vi "telem.vi"() -> ()   [LabVIEW 2015]
uses:
  <vilib>/Instr/_visa.llb/VISA Configure Serial Port (Instr).vi
panel:
  out "Heartbeat":bool
  in  "?":T1(tab)
  out "Pack voltage":u8(slide) scale=80.0..126.0
  out "Pack current":dbl format="%#_4gA"
  out "Max temperature":dbl format="%#_g°C"
  out "Pack voltage":dbl format="%#_5gV"
  out "Max voltage":dbl format="%#_4gV"
  out "Min voltage":dbl format="%#_4gV"
  in  "COM port":refnum<visa-resource-name>
  out "Battery status":bool
  out "Motor current":dbl format="%#_3fA"
  out "Battery status":bool
  out "Pack current":dbl format="%#_4gA"
  out "Temperature":u8[](array[numeric]) format="%d°C"
  out "Max temperature":dbl format="%#_g°C"
  out "Pack voltage":dbl format="%#_5gV"
  out "Max voltage":dbl format="%#_4gV"
  out "Min voltage":dbl format="%#_4gV"
  out "Voltage":u16[](array[slide]) scale=107.0..164.0
  out "Voltage":dbl[][](array[numeric]) format="%#_4gV"
  out "State of charge":dbl[][](array[numeric]) format="%#_4g%"
  out "Discharge":bool[](array[boolean])
  out "Motor power consumption":dbl format="%#_3fW"
  out "Gauge":dbl(knob) scale=0.0..100.0
  out "Motor velocity":dbl format="%#_7fkm/h"
  out "Bus voltage":dbl format="%#_3fV"
  out "Motor current":dbl format="%#_3fA"
  out "Motor rpm":dbl format="%#_10frpm"
  out "Motor internal temperature":dbl format="%#_3f°C"
  out "Motor heatsink temperature":dbl format="%#_3f°C"
  out "DSP board temperature":dbl format="%#_3f°C"
  out "Desired rpm":dbl format="%#_3frpm"
  out "Throttle":dbl format="%#_3f%"
  out "Array 1":bool[](array[boolean])
  out "Vin (1)":dbl format="%.2f"
  out "Vout (1)":dbl format="%.2f"
  out "Array 2":bool[](array[boolean])
  out "Array 3":bool[](array[boolean])
  out "Vin (3)":dbl format="%.2f"
  out "Vout (3)":dbl format="%.2f"
  out "Array 4":bool[](array[boolean])
  out "Vin (4)":dbl format="%.2f"
  out "Vout (4)":dbl format="%.2f"
  out "Iin (1)":dbl format="%.2f"
  out "Temperature (1)":u8
  out "Vin (2)":dbl
  out "Vout (2)":dbl format="%.2f"
  out "Iin (3)":dbl format="%.2f"
  out "Temperature (3)":u8
  out "Iin (4)":dbl format="%.2f"
  out "Temperature (4)":u8
  out "Iin (2)":dbl format="%.2f"
  out "Temperature (2)":u8
  out "Aux voltage":dbl
  out "DC/DC converter temperature":dbl format="%#_3g"
  out "Array connected":bool
  out "Motor connected":bool
  out "Aux cell voltages":dbl[][](array[numeric]) format="%#_4gV"
  out "0x0B - BPS voltage":string
  out "0x07 - Motor heatsink temperature":string
  out "0x05 - Motor velocity":string
  out "0x03 - Motor bus vi":string
  out "0x0D - BPS temperature":string
  out "0x11 - BPS current, balancing, status":string
  out "0x1D - MPPT":string
  out "0x09 - Motor DSP temperature":string
  out "0x19 - PMS data":string
  out "0x0A - EVDC drive":string
  # "1         2         3        4         5         6           7        8        9         10       11       12       13       14       15       16       17       18        19      20       21        22       23      24       25       26      27        28       29        30"
  # "UNDV  |  NOC   |  OVT  | BVLR"
  # "UNDV  |  NOC   |  OVT  | BVLR"
  # "UNDV  |  NOC   |  OVT  | BVLR"
  # "UNDV  |  NOC   |  OVT  | BVLR"
  # "Cell 1   |   Cell 2   |   Cell 3  |    Cell 4"
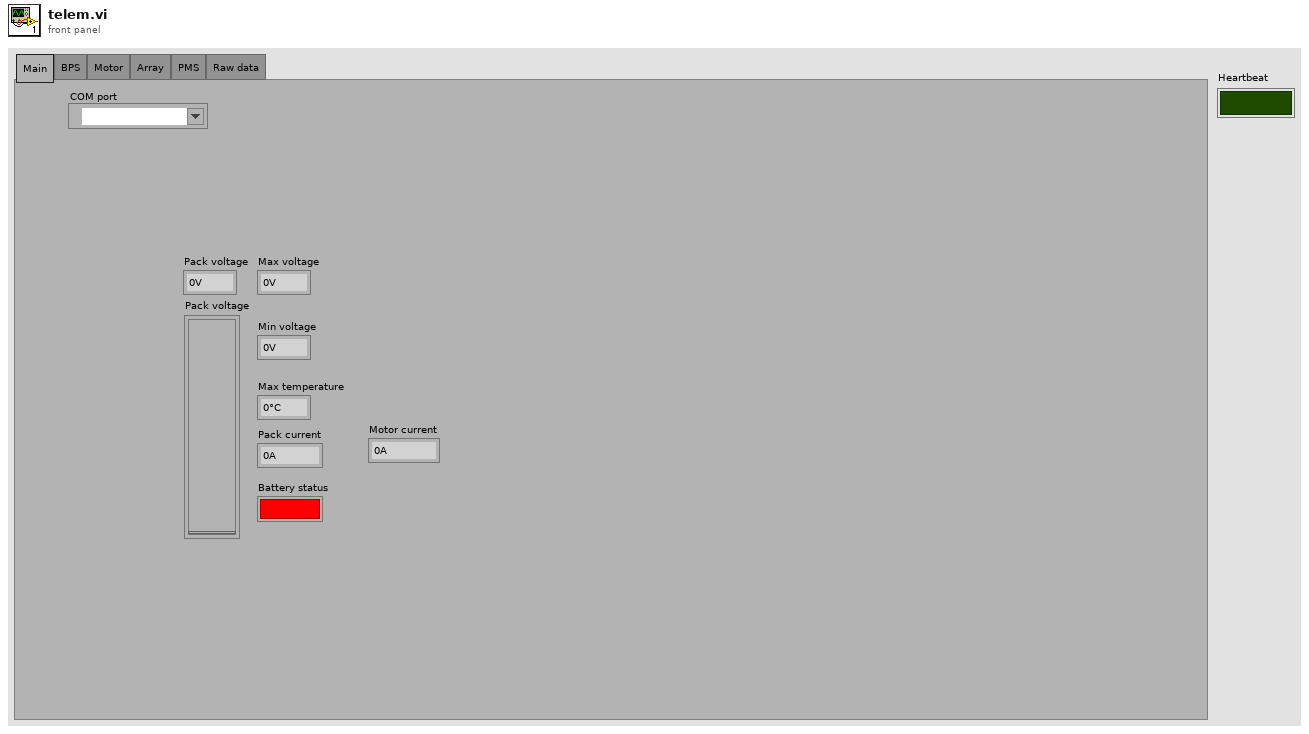
[diagram p1: front panel]
types:
  T1 = enum32{"Main", "BPS", "Motor", "Array", "PMS", "Raw data"}
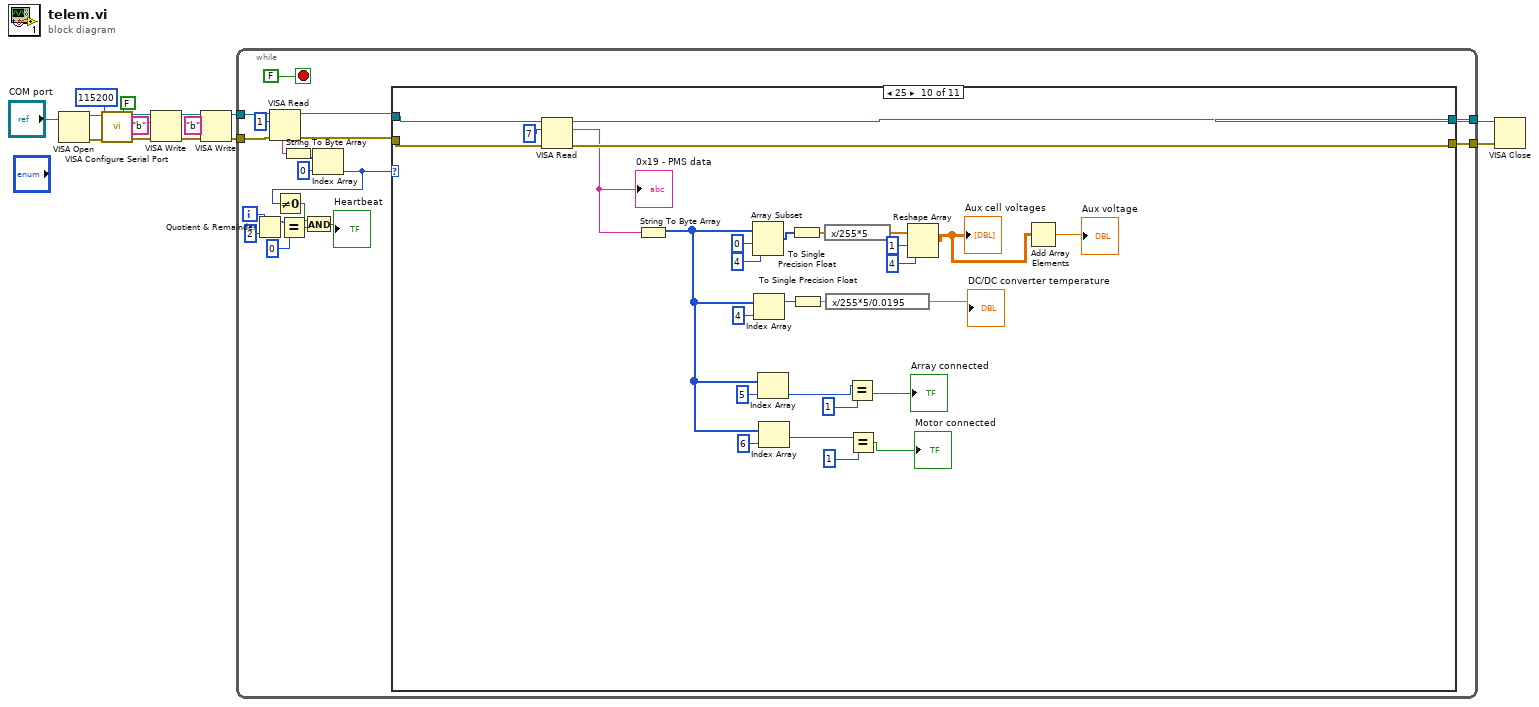
[diagram p0: block diagram]
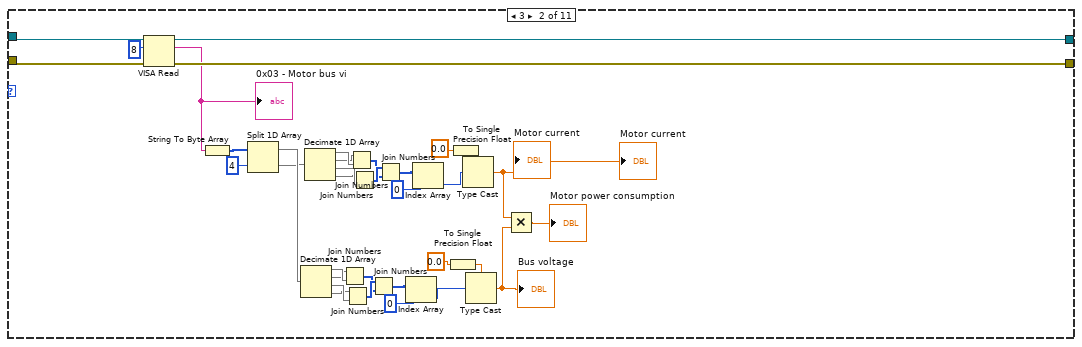
[diagram p3: hidden frame]
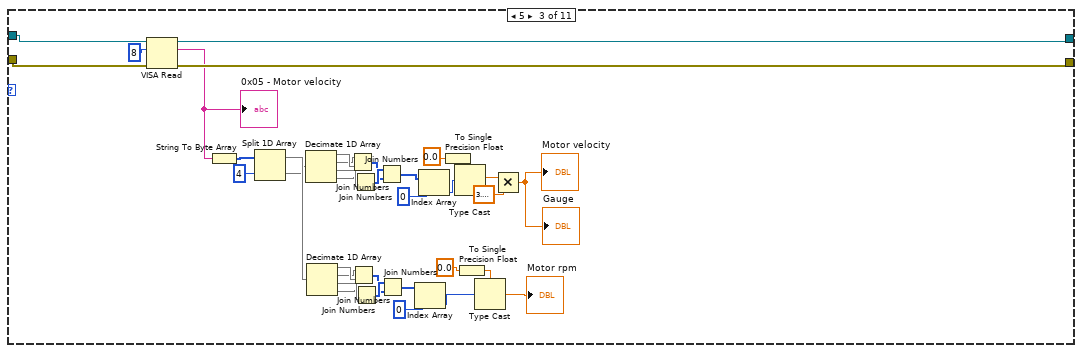
[diagram p4: hidden frame]
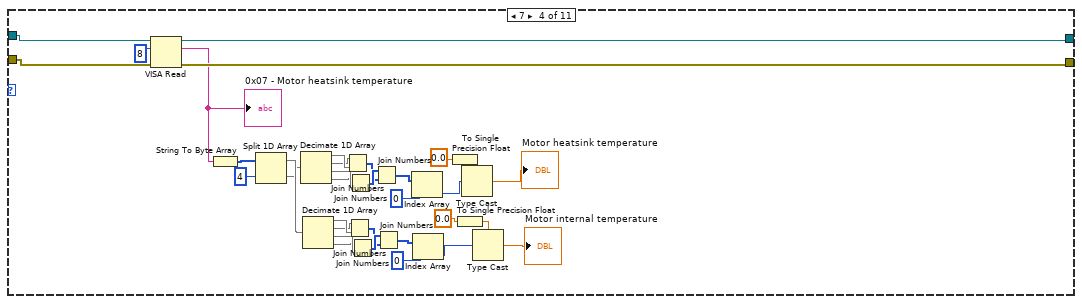
[diagram p5: hidden frame]
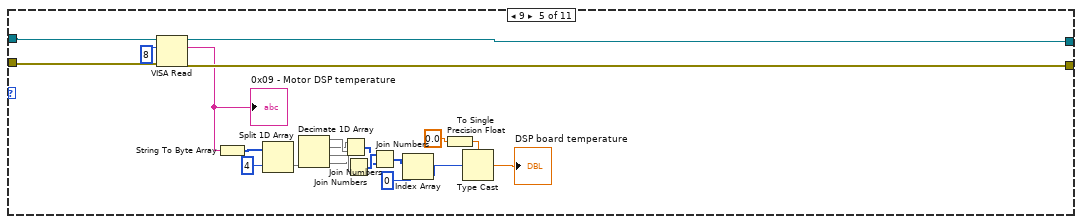
[diagram p6: hidden frame]
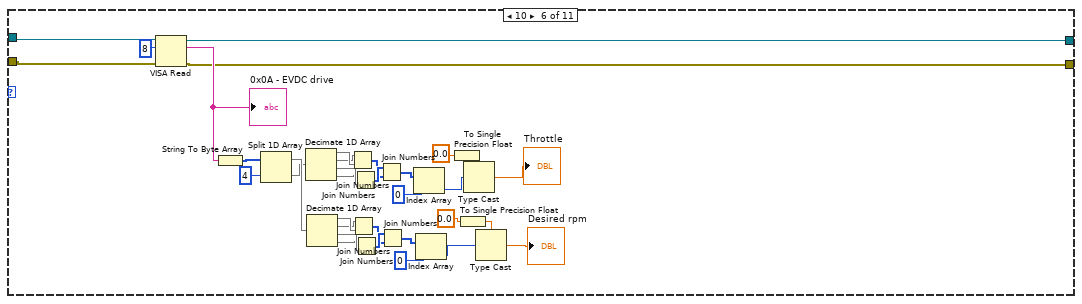
[diagram p7: hidden frame]
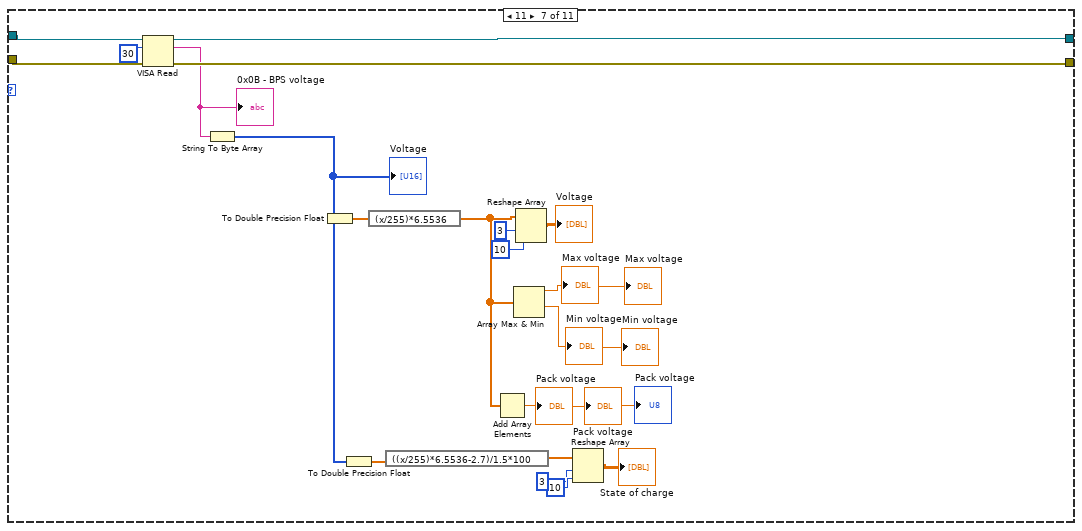
[diagram p8: hidden frame]
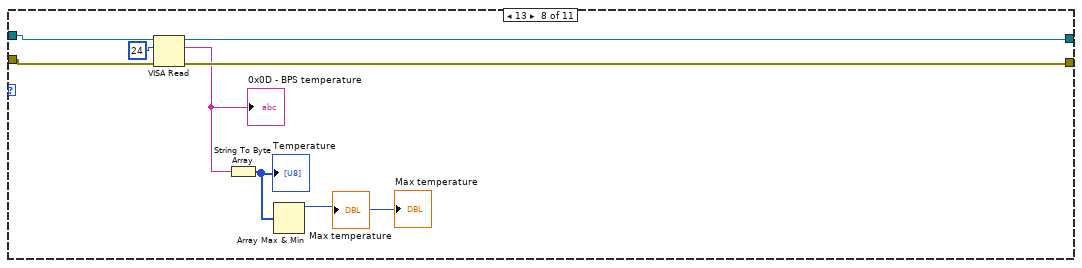
[diagram p9: hidden frame]
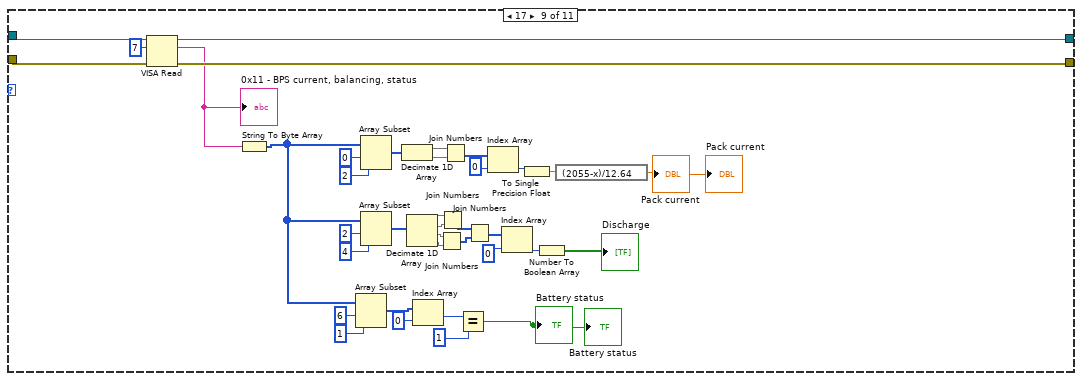
[diagram p10: hidden frame]
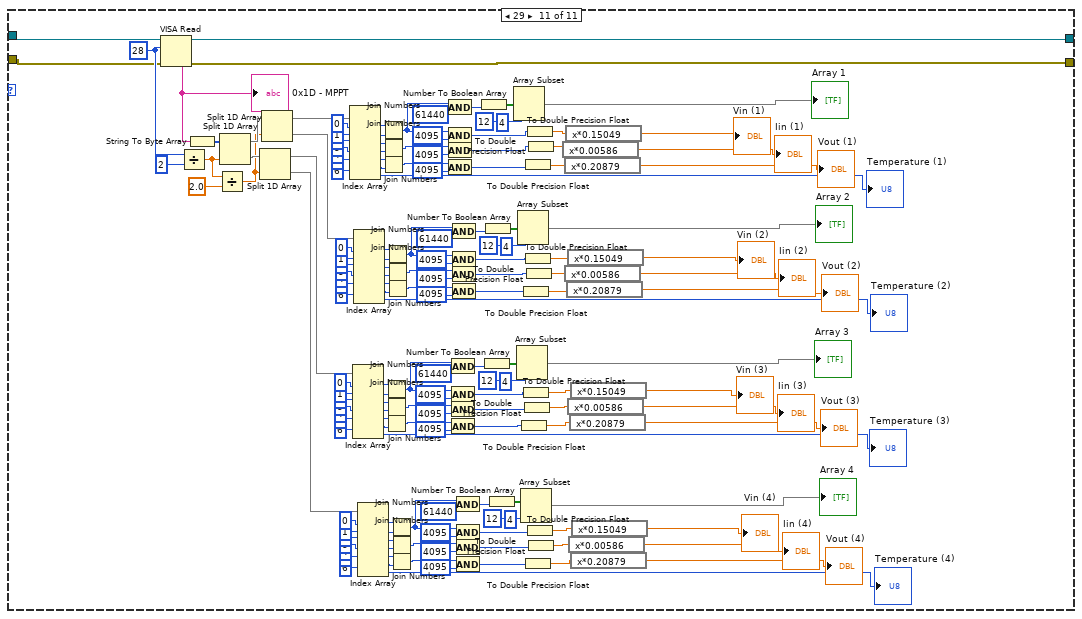
[diagram p11: hidden frame]
diagram:
  n1 = VISA Open(VISA resource name="COM port") -> (VISA resource name=w15:refnum<visa-resource-name>, error out=w14:errorcluster)  [unwired: 4 in]
  n2 = call-poly "VISA Configure Serial Port"("VISA resource name"=w15, "Enable Termination\nChar (T)"=FALSE ("Enable Termination\nChar (T)"), "baud rate (9600)"=u32 115200, "error in (no error)"=w14) -> ("VISA resource name out"=w8:refnum<visa-resource-name>, "error out"=w7:errorcluster)  [unwired: 10 in]
  n3 = VISA Write(VISA resource name=w8, write buffer="b", error in (no error)=w7) -> (VISA resource name out=w10:refnum<visa-resource-name>, error out=w9:errorcluster)  [unwired: 1 out]
  n4 = VISA Write(VISA resource name=w10, write buffer="b", error in (no error)=w9) -> (VISA resource name out=w3:refnum<visa-resource-name>, error out=w2:errorcluster)  [unwired: 1 out]
  n5 = while {
    tunnel: [w28] -> w5
    tunnel: [w27] -> w4
    tunnel: w3 -> [w17]
    tunnel: w2 -> [w16]
    i -> [w25]
    stop <- FALSE stop-if-true
    n6 = Quotient & Remainder(x=w25, y=2) -> (x-y*floor(x/y)=w23:i32)  [unwired: 1 out]
    n7 = VISA Read(VISA resource name=w17, byte count=u32 1, error in (no error)=w16) -> (VISA resource name out=w30:refnum<visa-resource-name>, read buffer=w33:string, error out=w29:errorcluster)  [unwired: 1 out]
    n8 = Equal?(x=w23, y=0) -> (x = y?=w21:bool)
    n9 = String To Byte Array(string=w33) -> (unsigned byte array=w32:u8[])
    n10 = Index Array(array=w32, index=0) -> (element=w18:u8)
    n11 = Not Equal To 0?(x=w18) -> (x != 0?=w20:bool)
    n12 = And(x=w20, y=w21) -> (x .and. y?=→"Heartbeat":bool)
    n13 = case shown="25" w18 {
      tunnel: w30 -> [w36 w53 w89 w125 w151 w180 w199 w218 w250 w286 w331]
      tunnel: w29 -> [w35 w52 w88 w124 w150 w179 w198 w217 w249 w285 w330]
      tunnel: [w36 w71 w107 w141 w162 w183 w216 w224 w261 w289 w446] -> w28
      tunnel: [w35 w70 w106 w140 w161 w182 w215 w223 w260 w288 w445] -> w27
      frame Default {
      }
      frame 3 {
        n14 = VISA Read(VISA resource name=w53, byte count=u32 8, error in (no error)=w52) -> (VISA resource name out=w71:refnum<visa-resource-name>, read buffer=w69:string, error out=w70:errorcluster)  [unwired: 1 out]
        "0x03 - Motor bus vi" <- w69
        n15 = String To Byte Array(string=w69) -> (unsigned byte array=w68:u8[])
        n16 = Split 1D Array(array=w68, index=4) -> (first subarray=w39:u8[], second subarray=w38:u8[])
        n17 = Decimate 1D Array(w39) -> (w41:u8[], w40:u8[], w43:u8[], w42:u8[])
        n18 = Decimate 1D Array(w38) -> (w51:u8[], w50:u8[], w49:u8[], w48:u8[])
        n19 = Join Numbers(hi=w40, lo=w41) -> ((hi.lo)=w44:u16[])
        n20 = Join Numbers(hi=w42, lo=w43) -> ((hi.lo)=w45:u16[])
        n21 = Join Numbers(hi=w50, lo=w51) -> ((hi.lo)=w46:u16[])
        n22 = Join Numbers(hi=w48, lo=w49) -> ((hi.lo)=w47:u16[])
        n23 = Join Numbers(hi=w45, lo=w44) -> ((hi.lo)=w64:u32[])
        n24 = Join Numbers(hi=w47, lo=w46) -> ((hi.lo)=w66:u32[])
        n25 = Index Array(array=w64, index=0) -> (element=w58:u32)
        n26 = Index Array(array=w66, index=0) -> (element=w62:u32)
        n27 = To Single Precision Float(number=sgl 0.0) -> (single precision float=w59:sgl)
        n28 = To Single Precision Float(number=sgl 0.0) -> (single precision float=w61:sgl)
        n29 = Type Cast(type=w61, x=w62) -> (*(type *) &x=w37:sgl)
        "Motor current" <- w37
        "Motor current" <- w37
        n30 = Type Cast(type=w59, x=w58) -> (*(type *) &x=w56:sgl)
        "Bus voltage" <- w56
        n31 = Multiply(x=w37, y=w56) -> (x*y=→"Motor power consumption":sgl)
      }
      frame 5 {
        n32 = VISA Read(VISA resource name=w89, byte count=u32 8, error in (no error)=w88) -> (VISA resource name out=w107:refnum<visa-resource-name>, read buffer=w94:string, error out=w106:errorcluster)  [unwired: 1 out]
        "0x05 - Motor velocity" <- w94
        n33 = String To Byte Array(string=w94) -> (unsigned byte array=w105:u8[])
        n34 = Split 1D Array(array=w105, index=4) -> (first subarray=w73:u8[], second subarray=w72:u8[])
        n35 = Decimate 1D Array(w72) -> (w87:u8[], w86:u8[], w85:u8[], w84:u8[])
        n36 = Decimate 1D Array(w73) -> (w81:u8[], w80:u8[], w79:u8[], w78:u8[])
        n37 = Join Numbers(hi=w86, lo=w87) -> ((hi.lo)=w82:u16[])
        n38 = Join Numbers(hi=w80, lo=w81) -> ((hi.lo)=w76:u16[])
        n39 = Join Numbers(hi=w84, lo=w85) -> ((hi.lo)=w83:u16[])
        n40 = Join Numbers(hi=w78, lo=w79) -> ((hi.lo)=w77:u16[])
        n41 = Join Numbers(hi=w83, lo=w82) -> ((hi.lo)=w74:u32[])
        n42 = Join Numbers(hi=w77, lo=w76) -> ((hi.lo)=w75:u32[])
        n43 = Index Array(array=w75, index=0) -> (element=w97:u32)
        n44 = Index Array(array=w74, index=0) -> (element=w101:u32)
        n45 = To Single Precision Float(number=sgl 0.0) -> (single precision float=w100:sgl)
        n46 = Type Cast(type=w100, x=w101) -> (*(type *) &x=w93:sgl)
        n47 = To Single Precision Float(number=sgl 0.0) -> (single precision float=w98:sgl)
        n48 = Type Cast(type=w98, x=w97) -> (*(type *) &x=→"Motor rpm":sgl)
        n49 = Multiply(x=w93, y=sgl 3.6) -> (x*y=→"Motor velocity" →"Gauge":sgl)
      }
      frame 7 {
        n50 = VISA Read(VISA resource name=w125, byte count=u32 8, error in (no error)=w124) -> (VISA resource name out=w141:refnum<visa-resource-name>, read buffer=w127:string, error out=w140:errorcluster)  [unwired: 1 out]
        "0x07 - Motor heatsink temperature" <- w127
        n51 = String To Byte Array(string=w127) -> (unsigned byte array=w139:u8[])
        n52 = Split 1D Array(array=w139, index=4) -> (first subarray=w109:u8[], second subarray=w108:u8[])
        n53 = Decimate 1D Array(w108) -> (w123:u8[], w122:u8[], w121:u8[], w120:u8[])
        n54 = Decimate 1D Array(w109) -> (w116:u8[], w115:u8[], w114:u8[], w113:u8[])
        n55 = Join Numbers(hi=w122, lo=w123) -> ((hi.lo)=w118:u16[])
        n56 = Join Numbers(hi=w115, lo=w116) -> ((hi.lo)=w111:u16[])
        n57 = Join Numbers(hi=w120, lo=w121) -> ((hi.lo)=w119:u16[])
        n58 = Join Numbers(hi=w113, lo=w114) -> ((hi.lo)=w112:u16[])
        n59 = Join Numbers(hi=w119, lo=w118) -> ((hi.lo)=w117:u32[])
        n60 = Join Numbers(hi=w112, lo=w111) -> ((hi.lo)=w110:u32[])
        n61 = Index Array(array=w117, index=0) -> (element=w135:u32)
        n62 = Index Array(array=w110, index=0) -> (element=w130:u32)
        n63 = To Single Precision Float(number=sgl 0.0) -> (single precision float=w133:sgl)
        n64 = To Single Precision Float(number=sgl 0.0) -> (single precision float=w131:sgl)
        n65 = Type Cast(type=w133, x=w135) -> (*(type *) &x=→"Motor heatsink temperature":sgl)
        n66 = Type Cast(type=w131, x=w130) -> (*(type *) &x=→"Motor internal temperature":sgl)
      }
      frame 9 {
        n67 = VISA Read(VISA resource name=w151, byte count=u32 8, error in (no error)=w150) -> (VISA resource name out=w162:refnum<visa-resource-name>, read buffer=w153:string, error out=w161:errorcluster)  [unwired: 1 out]
        "0x09 - Motor DSP temperature" <- w153
        n68 = String To Byte Array(string=w153) -> (unsigned byte array=w160:u8[])
        n69 = Split 1D Array(array=w160, index=4) -> (second subarray=w142:u8[])  [unwired: 1 out]
        n70 = Decimate 1D Array(w142) -> (w149:u8[], w148:u8[], w147:u8[], w146:u8[])
        n71 = Join Numbers(hi=w148, lo=w149) -> ((hi.lo)=w144:u16[])
        n72 = Join Numbers(hi=w146, lo=w147) -> ((hi.lo)=w145:u16[])
        n73 = Join Numbers(hi=w145, lo=w144) -> ((hi.lo)=w143:u32[])
        n74 = Index Array(array=w143, index=0) -> (element=w156:u32)
        n75 = To Single Precision Float(number=sgl 0.0) -> (single precision float=w157:sgl)
        n76 = Type Cast(type=w157, x=w156) -> (*(type *) &x=→"DSP board temperature":sgl)
      }
      frame 10 {
        n77 = VISA Read(VISA resource name=w180, byte count=u32 8, error in (no error)=w179) -> (VISA resource name out=w183:refnum<visa-resource-name>, read buffer=w184:string, error out=w182:errorcluster)  [unwired: 1 out]
        "0x0A - EVDC drive" <- w184
        n78 = String To Byte Array(string=w184) -> (unsigned byte array=w196:u8[])
        n79 = Split 1D Array(array=w196, index=4) -> (first subarray=w164:u8[], second subarray=w163:u8[])
        n80 = Decimate 1D Array(w163) -> (w178:u8[], w177:u8[], w176:u8[], w175:u8[])
        n81 = Decimate 1D Array(w164) -> (w172:u8[], w171:u8[], w170:u8[], w169:u8[])
        n82 = Join Numbers(hi=w177, lo=w178) -> ((hi.lo)=w173:u16[])
        n83 = Join Numbers(hi=w171, lo=w172) -> ((hi.lo)=w167:u16[])
        n84 = Join Numbers(hi=w175, lo=w176) -> ((hi.lo)=w174:u16[])
        n85 = Join Numbers(hi=w169, lo=w170) -> ((hi.lo)=w168:u16[])
        n86 = Join Numbers(hi=w174, lo=w173) -> ((hi.lo)=w165:u32[])
        n87 = Join Numbers(hi=w168, lo=w167) -> ((hi.lo)=w166:u32[])
        n88 = Index Array(array=w165, index=0) -> (element=w192:u32)
        n89 = Index Array(array=w166, index=0) -> (element=w187:u32)
        n90 = To Single Precision Float(number=sgl 0.0) -> (single precision float=w190:sgl)
        n91 = To Single Precision Float(number=sgl 0.0) -> (single precision float=w188:sgl)
        n92 = Type Cast(type=w190, x=w192) -> (*(type *) &x=→"Throttle":sgl)
        n93 = Type Cast(type=w188, x=w187) -> (*(type *) &x=→"Desired rpm":sgl)
      }
      frame 11 {
        n94 = VISA Read(VISA resource name=w199, byte count=u32 30, error in (no error)=w198) -> (VISA resource name out=w216:refnum<visa-resource-name>, read buffer=w204:string, error out=w215:errorcluster)  [unwired: 1 out]
        "0x0B - BPS voltage" <- w204
        n95 = String To Byte Array(string=w204) -> (unsigned byte array=w197:u8[])
        "Voltage" <- w197
        n96 = To Double Precision Float(number=w197) -> (double precision float=w214:dbl[])
        n97 = To Double Precision Float(number=w197) -> (double precision float=w213:dbl[])
        n98 = expression code="(x/255)*6.5536"(w214) -> (w205:dbl[])
        n99 = expression code="((x/255)*6.5536-2.7)/1.5*100"(w213) -> (w209:dbl[])
        n100 = Add Array Elements(numeric array=w205) -> (sum=→"Pack voltage" →"Pack voltage" →"Pack voltage":dbl)
        n101 = Array Max & Min(array=w205) -> (max value=→"Max voltage" →"Max voltage":dbl, min value=→"Min voltage" →"Min voltage":dbl)  [unwired: 2 out]
        n102 = Reshape Array(w205, 3 ("dimension size"), 10 ("dimension size")) -> (→"Voltage":dbl[][])
        n103 = Reshape Array(w209, 3 ("dimension size"), 10 ("dimension size")) -> (→"State of charge":dbl[][])
      }
      frame 13 {
        n104 = VISA Read(VISA resource name=w218, byte count=u32 24, error in (no error)=w217) -> (VISA resource name out=w224:refnum<visa-resource-name>, read buffer=w221:string, error out=w223:errorcluster)  [unwired: 1 out]
        "0x0D - BPS temperature" <- w221
        n105 = String To Byte Array(string=w221) -> (unsigned byte array=w222:u8[])
        "Temperature" <- w222
        n106 = Array Max & Min(array=w222) -> (max value=→"Max temperature" →"Max temperature":u8)  [unwired: 3 out]
      }
      frame 17 {
        n107 = VISA Read(VISA resource name=w250, byte count=u32 7, error in (no error)=w249) -> (VISA resource name out=w261:refnum<visa-resource-name>, read buffer=w255:string, error out=w260:errorcluster)  [unwired: 1 out]
        "0x11 - BPS current, balancing, status" <- w255
        n108 = String To Byte Array(string=w255) -> (unsigned byte array=w227:u8[])
        n109 = Array Subset(array=w227, index=6, length=1) -> (w229:u8[])
        n110 = Array Subset(array=w227, index=0, length=2) -> (w246:u8[])
        n111 = Array Subset(array=w227, index=2, length=4) -> (w234:u8[])
        n112 = Decimate 1D Array(w246) -> (w253:u8[], w252:u8[])
        n113 = Decimate 1D Array(w234) -> (w243:u8[], w242:u8[], w241:u8[], w240:u8[])
        n114 = Index Array(array=w229, index=0) -> (element=w233:u8)
        n115 = Join Numbers(hi=w241, lo=w240) -> ((hi.lo)=w239:u16[])
        n116 = Join Numbers(hi=w243, lo=w242) -> ((hi.lo)=w238:u16[])
        n117 = Join Numbers(hi=w253, lo=w252) -> ((hi.lo)=w258:u16[])
        n118 = Equal?(x=w233, y=u16 1) -> (x = y?=→"Battery status" →"Battery status":bool)
        n119 = Join Numbers(hi=w238, lo=w239) -> ((hi.lo)=w244:u32[])
        n120 = Index Array(array=w258, index=0) -> (element=w256:u16)
        n121 = Index Array(array=w244, index=0) -> (element=w245:u32)
        n122 = To Single Precision Float(number=w256) -> (single precision float=w257:sgl)
        n123 = Number To Boolean Array(number=w245) -> (Boolean array=→"Discharge":bool[])
        n124 = expression code="(2055-x)/12.64"(w257) -> (→"Pack current" →"Pack current":sgl)
      }
      frame 25 {
        n125 = VISA Read(VISA resource name=w286, byte count=u32 7, error in (no error)=w285) -> (VISA resource name out=w289:refnum<visa-resource-name>, read buffer=w284:string, error out=w288:errorcluster)  [unwired: 1 out]
        "0x19 - PMS data" <- w284
        n126 = String To Byte Array(string=w284) -> (unsigned byte array=w279:u8[])
        n127 = Array Subset(array=w279, index=0, length=4) -> (w267:u8[])
        n128 = Index Array(array=w279, index=4) -> (element=w265:u8)
        n129 = Index Array(array=w279, index=5) -> (element=w274:u8)
        n130 = Index Array(array=w279, index=6) -> (element=w276:u8)
        n131 = To Single Precision Float(number=w267) -> (single precision float=w268:sgl[])
        n132 = To Single Precision Float(number=w265) -> (single precision float=w266:sgl)
        n133 = expression code="x/255*5"(w268) -> (w269:sgl[])
        n134 = expression code="x/255*5/0.0195"(w266) -> (→"DC/DC converter temperature":sgl)
        n135 = Equal?(x=w274, y=u16 1) -> (x = y?=→"Array connected":bool)
        n136 = Equal?(x=w276, y=u16 1) -> (x = y?=→"Motor connected":bool)
        n137 = Reshape Array(w269, 1 ("dimension size"), 4 ("dimension size")) -> (w263:sgl[][])
        "Aux cell voltages" <- w263
        n138 = Add Array Elements(numeric array=w263) -> (sum=→"Aux voltage":sgl)
      }
      frame 29 {
        w332 = u32 28 ("byte count")
        n139 = VISA Read(VISA resource name=w331, byte count=w332, error in (no error)=w330) -> (VISA resource name out=w446:refnum<visa-resource-name>, read buffer=w444:string, error out=w445:errorcluster)  [unwired: 1 out]
        "0x1D - MPPT" <- w444
        n140 = Divide(x=w332, y=u8 2) -> (x/y=w431:dbl)
        n141 = String To Byte Array(string=w444) -> (unsigned byte array=w436:u8[])
        n142 = Divide(x=w431, y=2.0) -> (x/y=w432:dbl)
        n143 = Split 1D Array(array=w436, index=w431) -> (first subarray=w433:u8[], second subarray=w434:u8[])
        n144 = Split 1D Array(array=w434, index=w432) -> (first subarray=w334:u8[], second subarray=w333:u8[])
        n145 = Split 1D Array(array=w433, index=w432) -> (first subarray=w429:u8[], second subarray=w335:u8[])
        n146 = Index Array(array=w429, index #1=0 ("index"), index #2=1 ("index"), index #3=2 ("index"), index #4=3 ("index"), index #5=4 ("index"), index #6=5 ("index"), index #7=6 ("index")) -> (element #1=w427:u8, element #2=w428:u8, element #3=w416:u8, element #4=w415:u8, element #5=w412:u8, element #6=w411:u8, element #7=→"Temperature (1)":u8)
        n147 = Index Array(array=w334, index #1=0 ("index"), index #2=1 ("index"), index #3=2 ("index"), index #4=3 ("index"), index #5=4 ("index"), index #6=5 ("index"), index #7=6 ("index")) -> (element #1=w377:u8, element #2=w378:u8, element #3=w366:u8, element #4=w365:u8, element #5=w362:u8, element #6=w361:u8, element #7=→"Temperature (3)":u8)
        n148 = Index Array(array=w335, index #1=0 ("index"), index #2=1 ("index"), index #3=2 ("index"), index #4=3 ("index"), index #5=4 ("index"), index #6=5 ("index"), index #7=6 ("index")) -> (element #1=w402:u8, element #2=w403:u8, element #3=w391:u8, element #4=w390:u8, element #5=w387:u8, element #6=w386:u8, element #7=→"Temperature (2)":u8)
        n149 = Index Array(array=w333, index #1=0 ("index"), index #2=1 ("index"), index #3=2 ("index"), index #4=3 ("index"), index #5=4 ("index"), index #6=5 ("index"), index #7=6 ("index")) -> (element #1=w352:u8, element #2=w353:u8, element #3=w341:u8, element #4=w340:u8, element #5=w337:u8, element #6=w336:u8, element #7=→"Temperature (4)":u8)
        n150 = Join Numbers(hi=w427, lo=w428) -> ((hi.lo)=w420:u16)
        n151 = Join Numbers(hi=w416, lo=w415) -> ((hi.lo)=w418:u16)
        n152 = Join Numbers(hi=w412, lo=w411) -> ((hi.lo)=w414:u16)
        n153 = Join Numbers(hi=w377, lo=w378) -> ((hi.lo)=w370:u16)
        n154 = Join Numbers(hi=w366, lo=w365) -> ((hi.lo)=w368:u16)
        n155 = Join Numbers(hi=w362, lo=w361) -> ((hi.lo)=w364:u16)
        n156 = Join Numbers(hi=w402, lo=w403) -> ((hi.lo)=w395:u16)
        n157 = Join Numbers(hi=w391, lo=w390) -> ((hi.lo)=w393:u16)
        n158 = Join Numbers(hi=w387, lo=w386) -> ((hi.lo)=w389:u16)
        n159 = Join Numbers(hi=w352, lo=w353) -> ((hi.lo)=w345:u16)
        n160 = Join Numbers(hi=w341, lo=w340) -> ((hi.lo)=w343:u16)
        n161 = Join Numbers(hi=w337, lo=w336) -> ((hi.lo)=w339:u16)
        n162 = And(x=w420, y=u16 61440) -> (x .and. y?=w421:u16)
        n163 = And(x=w420, y=u16 4095) -> (x .and. y?=w299:u16)
        n164 = And(x=w418, y=u16 4095) -> (x .and. y?=w298:u16)
        n165 = And(x=w414, y=u16 4095) -> (x .and. y?=w297:u16)
        n166 = And(x=w370, y=u16 61440) -> (x .and. y?=w371:u16)
        n167 = And(x=w370, y=u16 4095) -> (x .and. y?=w300:u16)
        n168 = And(x=w368, y=u16 4095) -> (x .and. y?=w301:u16)
        n169 = And(x=w364, y=u16 4095) -> (x .and. y?=w302:u16)
        n170 = And(x=w395, y=u16 61440) -> (x .and. y?=w396:u16)
        n171 = And(x=w395, y=u16 4095) -> (x .and. y?=w296:u16)
        n172 = And(x=w393, y=u16 4095) -> (x .and. y?=w295:u16)
        n173 = And(x=w389, y=u16 4095) -> (x .and. y?=w294:u16)
        n174 = And(x=w345, y=u16 61440) -> (x .and. y?=w346:u16)
        n175 = And(x=w345, y=u16 4095) -> (x .and. y?=w311:u16)
        n176 = And(x=w343, y=u16 4095) -> (x .and. y?=w310:u16)
        n177 = And(x=w339, y=u16 4095) -> (x .and. y?=w309:u16)
        n178 = Number To Boolean Array(number=w421) -> (Boolean array=w425:bool[])
        n179 = Number To Boolean Array(number=w371) -> (Boolean array=w375:bool[])
        n180 = Number To Boolean Array(number=w396) -> (Boolean array=w400:bool[])
        n181 = Number To Boolean Array(number=w346) -> (Boolean array=w350:bool[])
        n182 = Array Subset(array=w425, index=12, length=4) -> (→"Array 1":bool[])
        n183 = Array Subset(array=w375, index=12, length=4) -> (→"Array 3":bool[])
        n184 = Array Subset(array=w400, index=12, length=4) -> (→"Array 2":bool[])
        n185 = To Double Precision Float(number=w302) -> (double precision float=w303:dbl)
        n186 = To Double Precision Float(number=w294) -> (double precision float=w291:dbl)
        n187 = To Double Precision Float(number=w300) -> (double precision float=w305:dbl)
        n188 = Array Subset(array=w350, index=12, length=4) -> (→"Array 4":bool[])
        n189 = To Double Precision Float(number=w301) -> (double precision float=w304:dbl)
        n190 = To Double Precision Float(number=w297) -> (double precision float=w312:dbl)
        n191 = To Double Precision Float(number=w296) -> (double precision float=w293:dbl)
        n192 = To Double Precision Float(number=w309) -> (double precision float=w308:dbl)
        n193 = To Double Precision Float(number=w295) -> (double precision float=w292:dbl)
        n194 = To Double Precision Float(number=w299) -> (double precision float=w314:dbl)
        n195 = To Double Precision Float(number=w311) -> (double precision float=w306:dbl)
        n196 = To Double Precision Float(number=w298) -> (double precision float=w313:dbl)
        n197 = To Double Precision Float(number=w310) -> (double precision float=w307:dbl)
        n198 = expression code="x*0.00586"(w313) -> (→"Iin (1)":dbl)
        n199 = expression code="x*0.20879"(w312) -> (→"Vout (1)":dbl)
        n200 = expression code="x*0.00586"(w292) -> (→"Iin (2)":dbl)
        n201 = expression code="x*0.15049"(w314) -> (→"Vin (1)":dbl)
        n202 = expression code="x*0.20879"(w291) -> (→"Vout (2)":dbl)
        n203 = expression code="x*0.15049"(w293) -> (→"Vin (2)":dbl)
        n204 = expression code="x*0.00586"(w304) -> (→"Iin (3)":dbl)
        n205 = expression code="x*0.00586"(w307) -> (→"Iin (4)":dbl)
        n206 = expression code="x*0.20879"(w303) -> (→"Vout (3)":dbl)
        n207 = expression code="x*0.15049"(w305) -> (→"Vin (3)":dbl)
        n208 = expression code="x*0.20879"(w308) -> (→"Vout (4)":dbl)
        n209 = expression code="x*0.15049"(w306) -> (→"Vin (4)":dbl)
      }
    }
  }
  n210 = VISA Close(VISA resource name=w5, error in (no error)=w4) -> ()  [unwired: 1 out]
